vi "Write Max Qorf DVR.vi"(8 "error in (no error)":errorcluster, 10 "Max Qorf DVR":refnum<data-value>, 11 "O3 Cal State in":refnum<class "O3 Cal State.lvclass">) -> (0 "error out":errorcluster, 3 "O3 Cal State out":refnum<class "O3 Cal State.lvclass">)   [LabVIEW 2012, in "O3 Cal State.lvclass"]
uses:
  O3 Cal State.lvclass
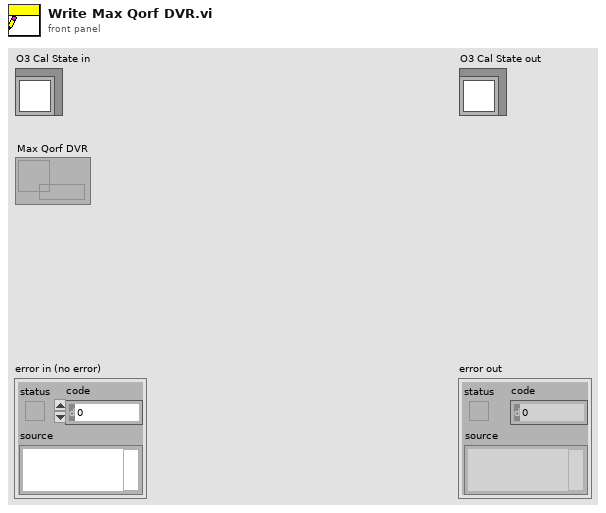
[diagram p1: front panel]
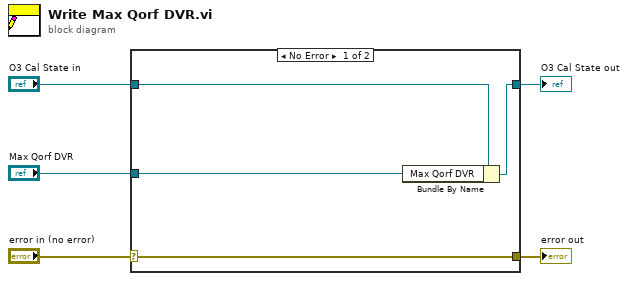
[diagram p0: block diagram]
diagram:
  n1 = case shown="No Error" "error in (no error)" {
    selector: "error in (no error)" -> [w9 w10]
    tunnel: [w9 w10] -> w4
    tunnel: [w7 w11] -> w2
    tunnel: "O3 Cal State in" -> [w8 w11]
    tunnel: "Max Qorf DVR" -> [w6 _]
    frame No Error {
      n2 = Bundle By Name(cluster=w8, "Max Qorf DVR"=w6) -> (w7:refnum<class "O3 Cal State.lvclass">)
    }
    frame Error {
    }
  }
  "error out" <- w4
  "O3 Cal State out" <- w2
